vi "Sub_Build_Fixed_Header.vi"(6 "Remaining Length":u32, 7 "Retain":T1, 8 "error in (no error)":errorcluster, 9 "QoS":T2, 10 "DUP":T3, 11 "MessageType":T4=enum."CONNECT") -> (0 "error out":errorcluster, 3 "Fixed Header":u8[](array[numeric]) format="%x")   [LabVIEW 2018, in "MQTT_Functions.lvlib"]
uses:
  MQTT_Functions.lvlib
  Controls/MessageType.ctl
  Controls/DUP_Flag.ctl
  Controls/QoS.ctl
  Controls/Retain_Flag.ctl
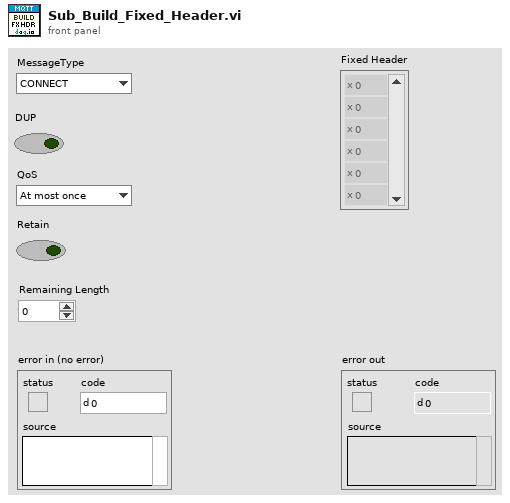
[diagram p1: front panel]
types:
  T1 = typedef "MQTT_Functions.lvlib/Retain_Flag.ctl" = bool
  T2 = typedef "MQTT_Functions.lvlib/QoS.ctl" = enum8{"At most once", "At least once", "Exactly once", "Reserved"}
  T3 = typedef "MQTT_Functions.lvlib/DUP_Flag.ctl" = bool
  T4 = typedef "MQTT_Functions.lvlib/MessageType.ctl" = enum32{"Reserved", "CONNECT", "CONNACK", "PUBLISH", "PUBACK", "PUBREC", "PUBREL", "PUBCOMP", "SUBSCRIBE", "SUBACK", "UNSUBSCRIBE", "UNSUBACK", "PINGREQ", "PINGRESP", "DISCONNECT", "Reserved2"}
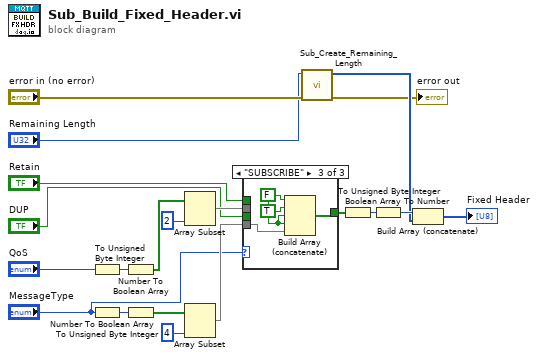
[diagram p0: block diagram]
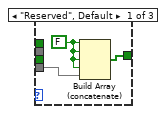
[diagram p2: hidden frame]
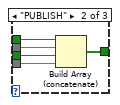
[diagram p3: hidden frame]
diagram:
  n1 = To Unsigned Byte Integer(number="QoS") -> (unsigned 8bit integer=w19:u8)
  n2 = To Unsigned Byte Integer(number="MessageType") -> (unsigned 8bit integer=w20:u8)
  n3 = Number To Boolean Array(number=w19) -> (Boolean array=w15:bool[])
  n4 = Number To Boolean Array(number=w20) -> (Boolean array=w17:bool[])
  n5 = Array Subset(array=w15, length=2) -> (w5:bool[])  [unwired: 1 in]
  n6 = Array Subset(array=w17, length=4) -> (w3:bool[])  [unwired: 1 in]
  n7 = case shown="\"SUBSCRIBE\"" "MessageType" {
    tunnel: [w23 w28 w29] -> w1
    tunnel: "Retain" -> [_ w27 _]
    tunnel: w5 -> [_ w26 _]
    tunnel: "DUP" -> [_ w25 _]
    tunnel: w3 -> [w21 w24 w32]
    frame "Reserved", Default {
      w22 = FALSE
      n8 = Build Array (concatenate)(w22, w22, w22, w22, w21) -> (w23:bool[])
    }
    frame "PUBLISH" {
      n9 = Build Array (concatenate)(w27, w26, w25, w24) -> (w28:T3[])
    }
    frame "SUBSCRIBE" {
      w30 = FALSE
      n10 = Build Array (concatenate)(w30, TRUE, w30, w30, w32) -> (w29:bool[])
    }
  }
  n11 = call "Sub_Create_Remaining_Length.vi"("error in (no error)"="error in (no error)", "X"="Remaining Length") -> ("error out"=→"error out":errorcluster, "bytes"=w11:u8[])  [unwired: 8 in]
  n12 = Boolean Array To Number(Boolean array=w1) -> (number=w13:u32)
  n13 = To Unsigned Byte Integer(number=w13) -> (unsigned 8bit integer=w12:u8)
  n14 = Build Array (concatenate)(w12, w11) -> (→"Fixed Header":u8[])
